vi "Request Config Info.vi"(8 "error in (no error)":errorcluster, 11 "SystemConfig MsgQ":refnum<class "MessageQ.lvclass">) -> (0 "error out":errorcluster, 2 "Config Info":T1, 3 "MessageQ":refnum<class "MessageQ.lvclass">)   [LabVIEW 2020, in "Volatus.lvlib"]
uses:
  Volatus.lvlib
  MessageQ/MessageQ.lvclass
  ConfigInfoValue/ConfigInfoValue.lvclass
  Config Info.ctl
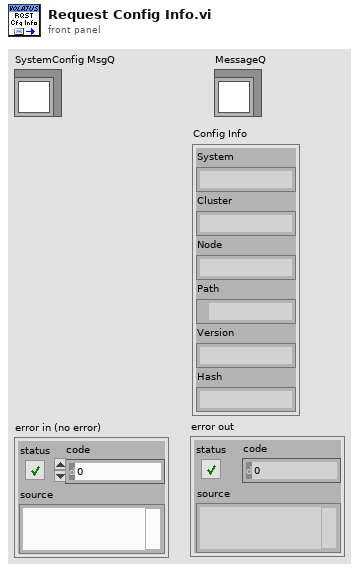
[diagram p1: front panel]
types:
  T1 = typedef "Volatus.lvlib/Config Info.ctl" = cluster{"System":string, "Cluster":string, "Node":string, "Path":path, "Version":string, "Hash":string}
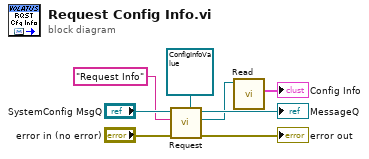
[diagram p0: block diagram]
diagram:
  n1 = call "Request.vi"("Response Type (None)"=refnum<class "ConfigInfoValue.lvclass"> refnum ("Volatus:ConfigInfoValue.lvclass"), "error in (no error)"="error in (no error)", "ID"="Request Info", "MessageQ in"="SystemConfig MsgQ") -> ("error out"=→"error out":errorcluster, "Response"=w2:refnum<class "ConfigInfoValue.lvclass">, "MessageQ out"=→"MessageQ":refnum<class "MessageQ.lvclass">)  [unwired: 5 in]
  n2 = call "Read.vi"("ConfigInfoValue in"=w2) -> ("Config Info"=→"Config Info":T1)  [unwired: 10 in]
